vi "Once.vi"(1 "Reset?":bool, 2 "Input":bool) -> (0 "Output":bool)   [LabVIEW 2012]
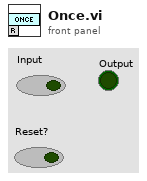
[diagram p1: front panel]
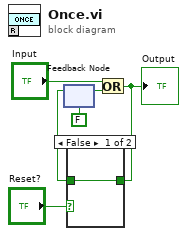
[diagram p0: block diagram]
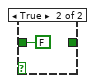
[diagram p2: hidden frame]
diagram:
  n1 = feedback #1(FALSE) -> (w5:bool)
  n2 = Or(x="Input", y=w5) -> (x .or. y?=w3:bool)
  "Output" <- w3
  n3 = case shown="False" "Reset?" {
    tunnel: w3 -> [w7 _]
    tunnel: [w7 FALSE] -> w2
    frame False {
    }
    frame True {
    }
  }
  n4 = feedback-in #1(w2) -> ()
